vi "sample_withref.vi"() -> ()   [LabVIEW 2013]
panel:
  out "x/y":dbl
  out "next step":dbl
  in  "0,01":T1={"X-Abstand (0)"=0.0, "Y-Abstand (0)"=0.01, "Z-Abstand (0)"=0.0}
  in  "speed 0,01":T2={"Startgeschwindigkeit\nin mm/s (10) [0,1-150]"=10.0, "Sollgeschwindigkeit\nin mm/s (10) [0,1-150]"=0.5, "Stopgeschwindigkeit\nin mm/s (10) [0,1-150]"=10.0}
  in  "Richtungen":T3 {"Richtung Z (vEw)" items=["vom Endschalter weg", "zum Endschalter hin"]; "Richtung Y (vEw)" items=["vom Endschalter weg", "zum Endschalter hin"]; "Richtung X (vEw)" items=["vom Endschalter weg", "zum Endschalter hin"]}
  in  "4,9":T1={"X-Abstand (0)"=0.0, "Y-Abstand (0)"=4.9, "Z-Abstand (0)"=0.0}
  in  "speed 4,9":T2={"Startgeschwindigkeit\nin mm/s (10) [0,1-150]"=10.0, "Sollgeschwindigkeit\nin mm/s (10) [0,1-150]"=5.0, "Stopgeschwindigkeit\nin mm/s (10) [0,1-150]"=10.0}
  out "ED33_output":string[][](array[string])
  out "Koordinaten IF6":T4 {"Schritte B" format="%#.4g"; "Schritte A" format="%#.4g"; "Schritte C" format="%#.4g"; "Schritte U" format="%#.4g"; "Schritte Z" format="%#.4g"; "Schritte Y" format="%#.4g"; "Schritte X" format="%#.4g"}
  out "Diff":i64
  out "ref":i64
  out "new_pos":i64
  out "pos":i64
  out "VISA resource name out":refnum<visa-resource-name>
  in  "Port Kosy":refnum<visa-resource-name>="COM2"
  out "error out":errorcluster
  in  "error in":errorcluster
  out "element":string
  out "subarray":string[](array[string])
  in  "Port ED33":refnum<visa-resource-name>="COM7"
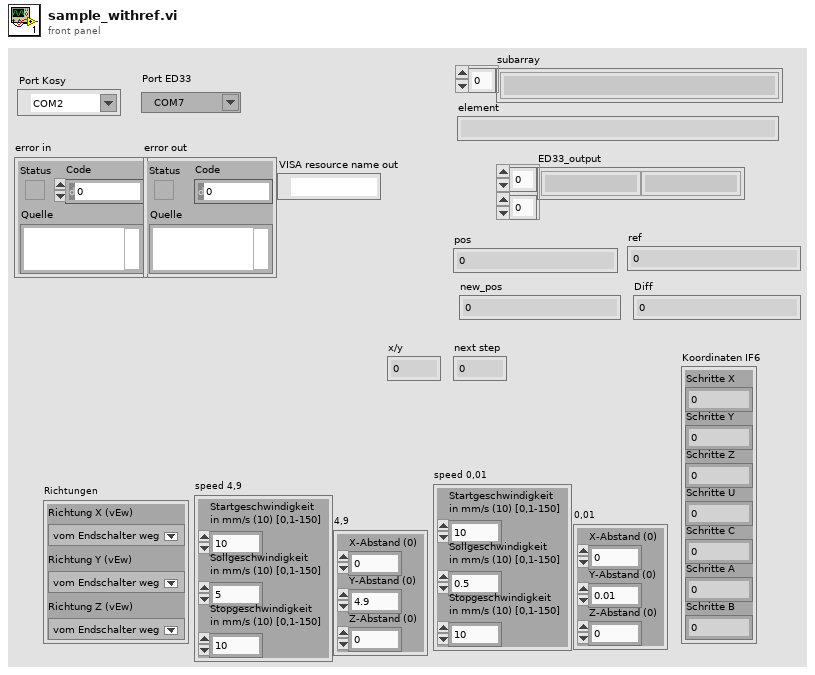
[diagram p1: front panel]
types:
  T1 = cluster{"X-Abstand (0)":sgl, "Y-Abstand (0)":sgl, "Z-Abstand (0)":sgl}
  T2 = cluster{"Startgeschwindigkeit\nin mm/s (10) [0,1-150]":sgl, "Sollgeschwindigkeit\nin mm/s (10) [0,1-150]":sgl, "Stopgeschwindigkeit\nin mm/s (10) [0,1-150]":sgl}
  T3 = cluster{"Richtung X (vEw)":u16, "Richtung Y (vEw)":u16, "Richtung Z (vEw)":u16}
  T4 = cluster{"Schritte X":sgl, "Schritte Y":sgl, "Schritte Z":sgl, "Schritte U":sgl, "Schritte C":sgl, "Schritte A":sgl, "Schritte B":sgl}
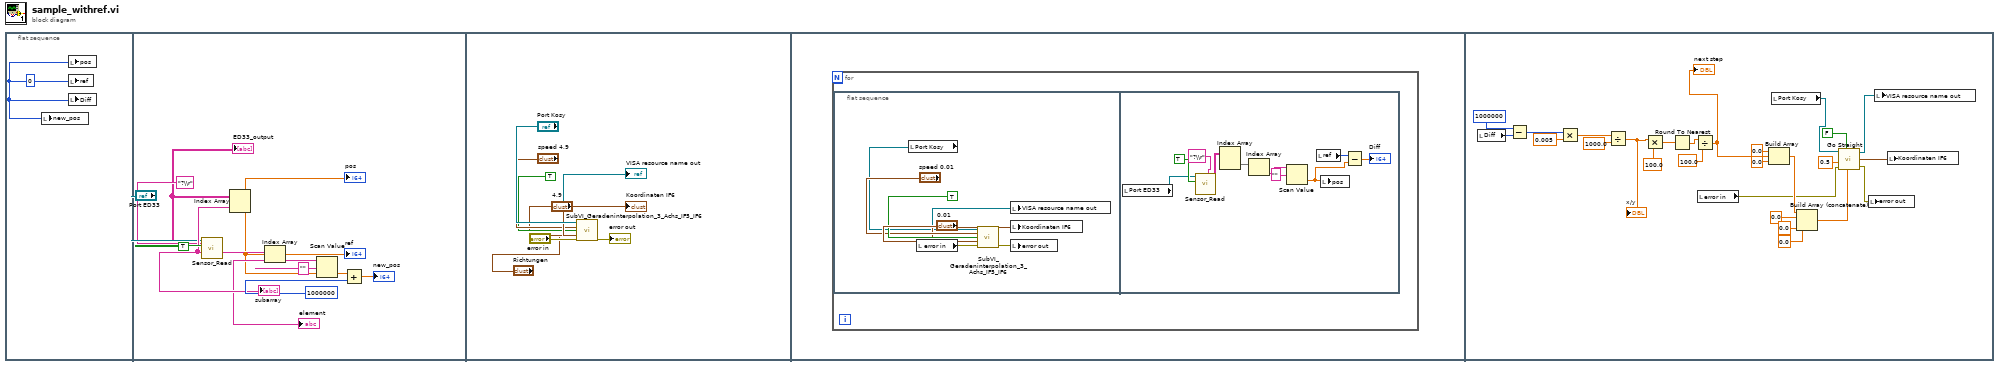
[diagram p0: block diagram]
diagram:
  n1 = flat-sequence {
    frame #0 {
      w1 = i64 0 ("pos")
      n2 = local write "new_pos"(w1) -> ()
      n3 = local write "pos"(w1) -> ()
      n4 = local write "ref"(w1) -> ()
      n5 = local write "Diff"(w1) -> ()
    }
    frame #1 {
      n6 = call "Sensor_Read.vi"("write ED33"="?\\r", "ED33 Active?"=TRUE, "Port ED33"="Port ED33") -> ("ED33_output"=w2:string[][])  [unwired: 7 in, 1 out]
      "ED33_output" <- w2
      n7 = Index Array(array=w2) -> (element=w8:string[])  [unwired: 2 in]
      "subarray" <- w8
      n8 = Index Array(array=w8) -> (element=w6:string)  [unwired: 1 in]
      "element" <- w6
      n9 = Scan Value(string=w6, format string="") -> (value=w5:dbl)  [unwired: 1 in, 1 out]
      "pos" <- w5
      "ref" <- w5
      n10 = Add(x=w5, y=1000000) -> (x+y=→"new_pos":dbl)
    }
    frame #2 {
      n11 = call <userlib>:"SubVI_Geradeninterpolation_3_Achs_IF5_IF6.vi"("VISA resource name in"="Port Kosy", "Geschwindigkeiten"="speed 4,9", "IF5=F/IF6=T\n(IF6=T) in"=TRUE ("IF5=F/IF6=T\n(IF6=T) in"), "Abstände"="4,9", "error in"="error in", "Richtungen"="Richtungen") -> ("VISA resource name out"=→"VISA resource name out":refnum<visa-resource-name>, "Koordinaten IF6"=→"Koordinaten IF6":T4, "error out"=→"error out":errorcluster)  [unwired: 4 in, 3 out]
    }
    frame #3 {
      n12 = for {
        N: 8 -> [_]
        n13 = flat-sequence {
          frame #0 {
            n14 = local read "Port Kosy"() -> (w22:refnum<visa-resource-name>)
            n15 = local read "error in"() -> (w26:errorcluster)
            n16 = call <userlib>:"SubVI_Geradeninterpolation_3_Achs_IF5_IF6.vi"("VISA resource name in"=w22, "Geschwindigkeiten"="speed 0,01", "IF5=F/IF6=T\n(IF6=T) in"=TRUE ("IF5=F/IF6=T\n(IF6=T) in"), "Abstände"="0,01", "error in"=w26) -> ("VISA resource name out"=w23:refnum<visa-resource-name>, "Koordinaten IF6"=w24:T4, "error out"=w25:errorcluster)  [unwired: 5 in, 3 out]
            n17 = local write "VISA resource name out"(w23) -> ()
            n18 = local write "Koordinaten IF6"(w24) -> ()
            n19 = local write "error out"(w25) -> ()
          }
          frame #1 {
            n20 = local read "Port ED33"() -> (w32:refnum<visa-resource-name>)
            n21 = call "Sensor_Read.vi"("write ED33"="?\\r", "ED33 Active?"=TRUE, "Port ED33"=w32) -> ("ED33_output"=w34:string[][])  [unwired: 7 in, 1 out]
            n22 = Index Array(array=w34) -> (element=w35:string[])  [unwired: 2 in]
            n23 = Index Array(array=w35) -> (element=w30:string)  [unwired: 1 in]
            n24 = Scan Value(string=w30, format string="") -> (value=w38:dbl)  [unwired: 1 in, 1 out]
            n25 = local read "ref"() -> (w37:i64)
            n26 = local write "pos"(w38) -> ()
            n27 = Subtract(x=w37, y=w38) -> (x-y=→"Diff":dbl)
          }
        }
      }
    }
    frame #4 {
      n28 = local read "Diff"() -> (w65:i64)
      n29 = Subtract(x=i64 1000000, y=w65) -> (x-y=w63:i64)
      n30 = Multiply(x=w63, y=0.005) -> (x*y=w62:dbl)
      n31 = Divide(x=w62, y=1000.0) -> (x/y=w59:dbl)
      "x/y" <- w59
      n32 = Multiply(x=w59, y=100.0) -> (x*y=w57:dbl)
      n33 = Round To Nearest(number=w57) -> (nearest integer value=w56:dbl)
      n34 = Divide(x=w56, y=100.0) -> (x/y=w51:dbl)
      "next step" <- w51
      n35 = local read "error in"() -> (w40:errorcluster)
      n36 = Build Array(0.0 ("element"), w51, 0.0 ("element")) -> (w48:dbl[])
      n37 = local read "Port Kosy"() -> (w43:refnum<visa-resource-name>)
      n38 = Build Array (concatenate)(w48, 0.0 ("element"), 0.0 ("element"), 0.0 ("element")) -> (w47:dbl[])
      n39 = call "Go Straight.vi"("VISA resource name in"=w43, "Sequence Active"=FALSE, "Speed"=0.5, "Steps(mm)"=w47, "error in"=w40) -> ("VISA resource name out"=w42:refnum<visa-resource-name>, "Koordinaten IF6"=w44:T4, "error out"=w41:errorcluster)  [unwired: 1 in]
      n40 = local write "error out"(w41) -> ()
      n41 = local write "VISA resource name out"(w42) -> ()
      n42 = local write "Koordinaten IF6"(w44) -> ()
    }
  }
